vi "DAQ-damon.vi"(10 "Parameters":T1, 11 "queue out":refnum<queue>) -> ()   [LabVIEW 2014]
uses:
  Controls/FGVisfileopen.ctl
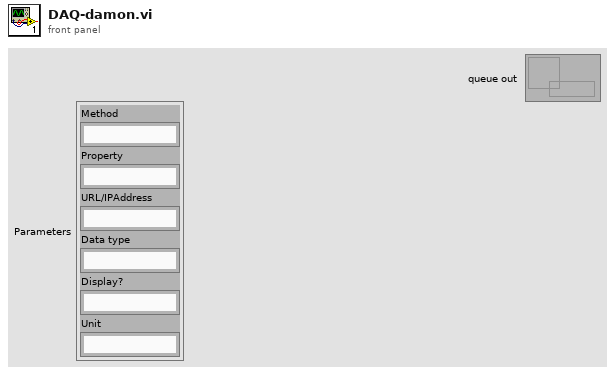
[diagram p1: front panel]
types:
  T1 = cluster{"Method":string, "Property":string, "URL/IPAddress":string, "Data type":string, "Display?":string, "Unit":string}
  T2 = typedef "FGVisfileopen.ctl" = enum16{"Read", "Write"}
  T3 = cluster{"Method":string, "PropertyName":string, "Value":string, "Display?":string, "Unit":string}
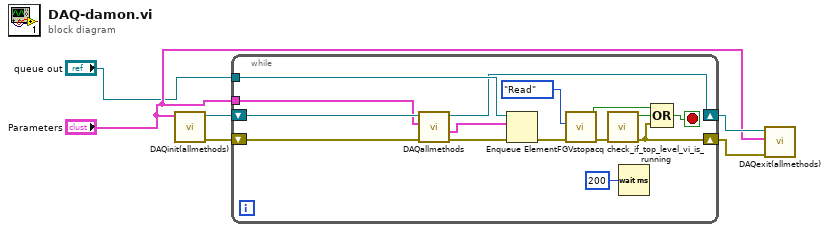
[diagram p0: block diagram]
diagram:
  n1 = call "DAQinit(allmethods).vi"("Parameters"="Parameters") -> ("error out"=w3:errorcluster, "INITout"=w4:refnum<class "RADEBase.lvclass">)  [unwired: 9 in]
  n2 = while {
    tunnel: "queue out" -> [w17]
    shift-right: [w15] -> w6
    shift-left: w4 -> [w16]
    shift-right: [w13] -> w5
    shift-left: w3 -> [w9]
    tunnel: "Parameters" -> [w10]
    stop <- w19 stop-if-true
    n3 = call "DAQallmethods.vi"("error in"=w9, "Parameters"=w10, "fromINIT"=w16) -> ("error out"=w14:errorcluster, "Data Pack"=w7:T3, "toExit"=w15:refnum<class "RADEBase.lvclass">)  [unwired: 6 in]
    n4 = Enqueue Element(queue=w17, element=w7, error in (no error)=w14) -> (error out=w12:errorcluster)  [unwired: 1 in, 2 out]
    n5 = call "FGVstopacq.vi"("error in"=w12, "Write from FGV or Read from FGV?"=FGVisfileopen."Read") -> ("error out"=w20:errorcluster, "Output Value"=w11:bool)  [unwired: 8 in]
    n6 = call "check_if_top_level_vi_is_running.vi"("error in (no error)"=w20) -> ("error out"=w13:errorcluster, "stop?"=w18:bool)  [unwired: 9 in]
    n7 = Wait (ms)(milliseconds to wait=u32 200) -> ()  [unwired: 1 out]
    n8 = Compound Arithmetic op=OR(w11, w18, w13) -> (w19:bool)
  }
  n9 = call "DAQexit(allmethods).vi"("error in"=w5, "Parameters"="Parameters", "INITout"=w6) -> ()  [unwired: 8 in, 1 out]
